vi "Frame Calc Wrapper.vi"() -> (5 "Frames/s received":dbl)   [LabVIEW 2021, in "DecodetoImage.lvlib"]
uses:
  DecodetoImage.lvlib
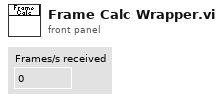
[diagram p1: front panel]
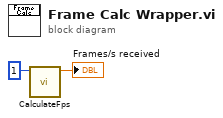
[diagram p0: block diagram]
diagram:
  n1 = call "CalculateFps.vi"("New Frames Transferred"=u64 1) -> ("Frames/s"=→"Frames/s received":dbl)  [unwired: 10 in]
